vi "UpdateMDF.vi"(8 "Index":i32, 11 "MDF In":T1[](array[typedef])) -> (3 "MDF Out":T1[](array[typedef]))   [LabVIEW 2011]
doc: "This VI updates the status control in the MDF cluster"
uses:
  MDF.ctl
  Behaviour.ctl
panel:
  out "MDF_Out":T3(array[cluster])
  in  "MDF_In":T3(array[cluster])
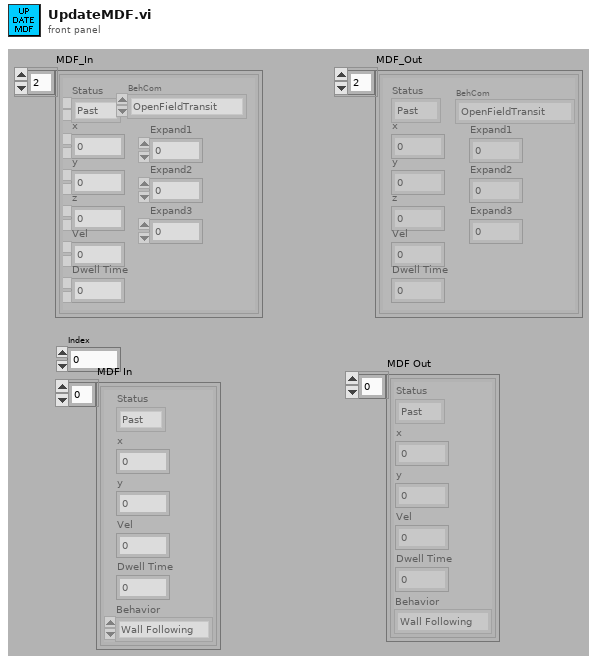
[diagram p1: front panel]
types:
  T1 = typedef "MDF.ctl" = cluster{"Status":enum16{"Past", "Current", "Future"}, "x":dbl, "y":dbl, "Vel":dbl, "Dwell Time":dbl, "Behavior":T2}
  T2 = typedef "Behaviour.ctl" = enum16{"Wall Following", "Open Transit", "Find Barge", "Push Barge", "Go Home"}
  T3 = cluster{"Status":enum16{"Past", "Current", "Future"}, "x":dbl, "y":dbl, "z":dbl, "Vel":dbl, "Dwell Time":dbl, "BehCom":enum16{"OpenFieldTransit", "P-WallFollow", "S-WallFollow", "LaneFollow", "ManualMode"}, "Expand1":dbl, "Expand2":dbl, "Expand3":dbl}[]
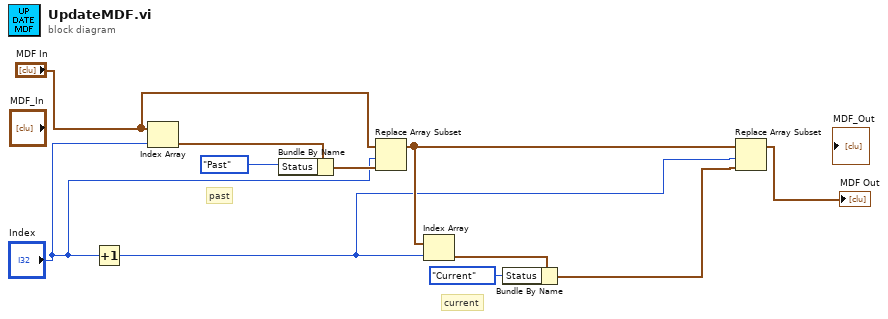
[diagram p0: block diagram]
diagram:
  # "current"
  # "past"
  n1 = Increment(x="Index") -> (x+1=w3:i32)
  n2 = Index Array "Index Array"(array="MDF In", index="Index") -> (element=w11:T1)
  n3 = Bundle By Name(cluster=w11, "Status"=enum16{"Past", "Current", "Future"}."Past") -> (w10:T1)
  n4 = Replace Array Subset "Replace Array Subset"(array="MDF In", new element=w10, index="Index") -> (w7:T1[])
  n5 = Index Array "Index Array"(array=w7, index=w3) -> (element=w6:T1)
  n6 = Bundle By Name(cluster=w6, "Status"=enum16{"Past", "Current", "Future"}."Current") -> (w4:T1)
  n7 = Replace Array Subset "Replace Array Subset"(array=w7, new element=w4, index=w3) -> (→"MDF Out":T1[])
